vi "Simulation Interface.vi"(8 "error in (no error)":errorcluster, 11 "View Model":T1) -> (0 "error out":errorcluster)   [LabVIEW 2017]
doc: "A program that is run to test Elevator algorithms in a SW-only environment."
uses:
  View Model/Controls/View Model.ctl
  View Model/Controls/Shared Model.ctl
  Error/Controls/Error Model.ctl
  Error/Controls/Error Event.ctl
  Error/Controls/Error Type.ctl
  Configuration/Controls/Config DB Model.ctl
  Configuration/Controls/Config DB Command.ctl
  Configuration/Controls/Config DB Record.ctl
  Controller/Controls/Controller Model.ctl
  Controller/Controls/Elevator Location.ctl
  Controller/Controls/Elevator Direction Event.ctl
  Controller/Controls/Elevator Direction.ctl
  Controller/Controls/Elevator CMD Event.ctl
  Controller/Controls/Elevator Commands.ctl
  Controller/Controls/Elevator Overhead.ctl
  Controller/Controls/Elevator State.ctl
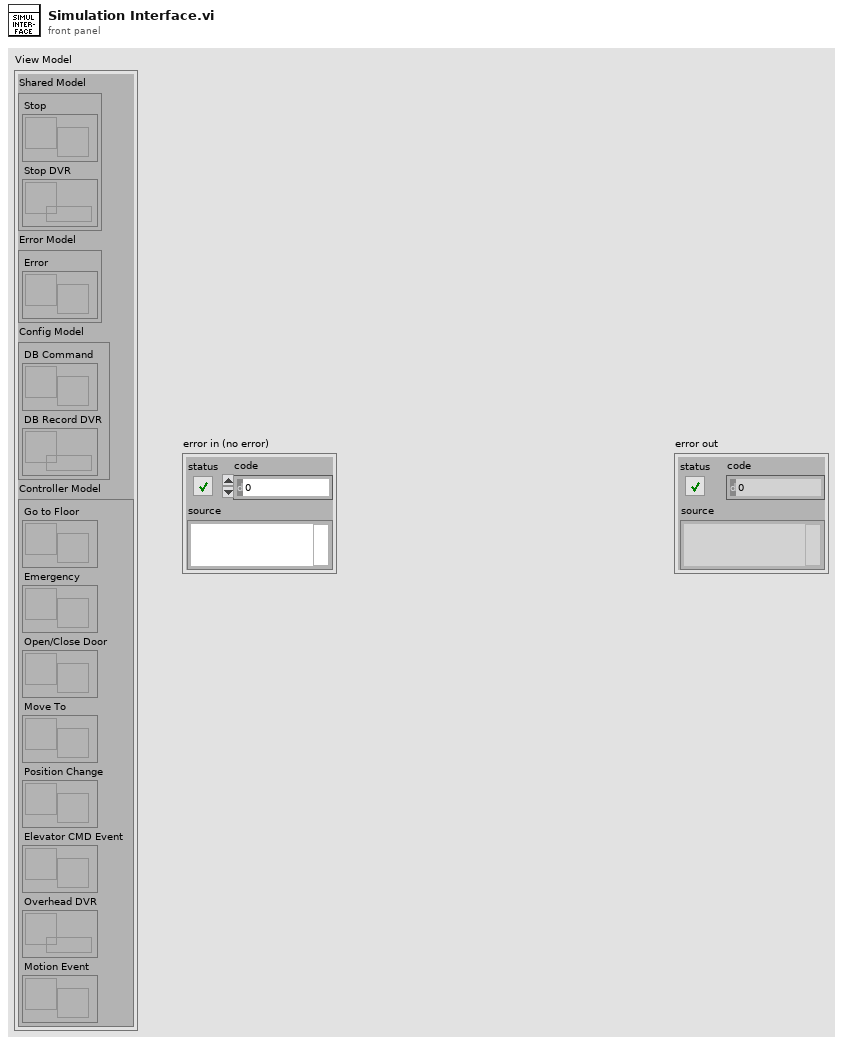
[diagram p1: front panel]
types:
  T1 = typedef "View Model.ctl" = cluster{"Shared Model":T2, "Error Model":T3, "Config Model":T4, "Controller Model":T5}
  T2 = typedef "Shared Model.ctl" = cluster{"Stop":refnum<user-event>, "Stop DVR":refnum<data-value>}
  T3 = typedef "Error Model.ctl" = cluster{"Error":refnum<user-event>}
  T4 = typedef "Config DB Model.ctl" = cluster{"DB Command":refnum<user-event>, "DB Record DVR":refnum<data-value>}
  T5 = typedef "Controller Model.ctl" = cluster{"Go to Floor":refnum<user-event>, "Emergency":refnum<user-event>, "Open/Close Door":refnum<user-event>, "Move To":refnum<user-event>, "Position Change":refnum<user-event>, "Elevator CMD Event":refnum<user-event>, "Overhead DVR":refnum<data-value>, "Motion Event":refnum<user-event>}
  T6 = enum32{"invalid app kind", "Development System", "Run Time System", "Student Edition", "Embedded LabVIEW", "Evaluation", "Custom"}
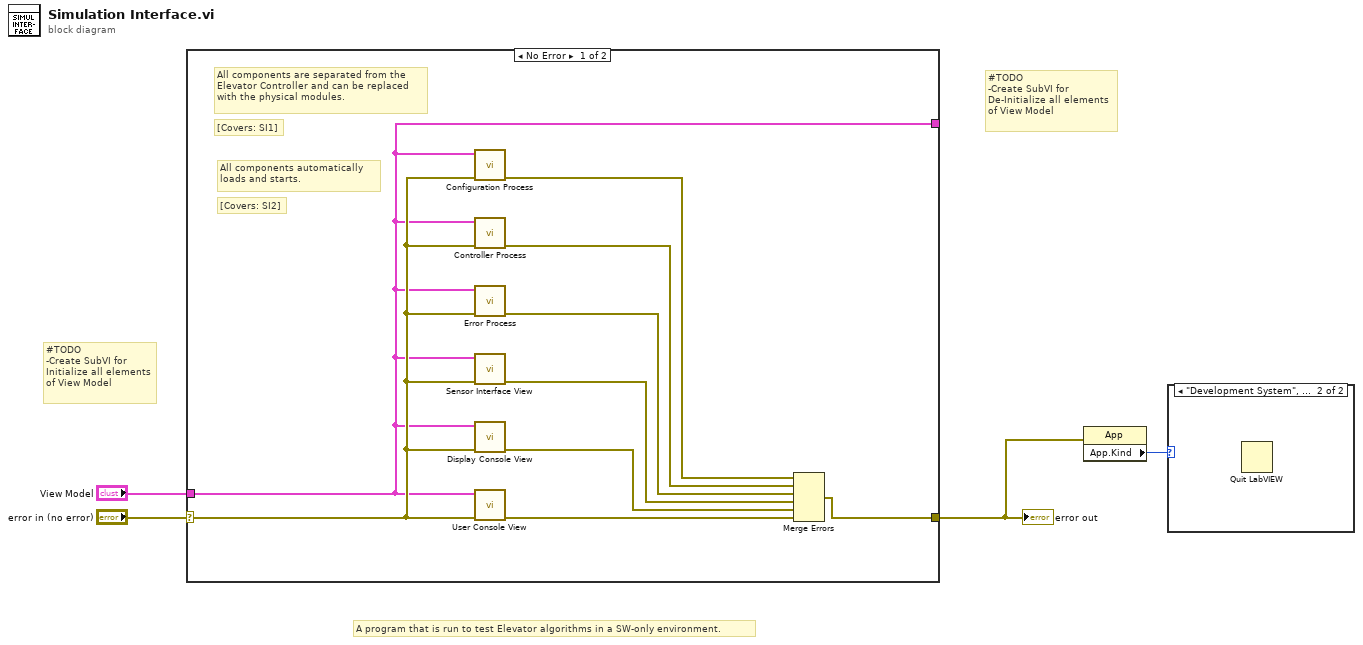
[diagram p0: block diagram]
diagram:
  # "#TODO\n-Create SubVI for\nDe-Initialize all elements\nof View Model"
  # "#TODO\n-Create SubVI for\nInitialize all elements\nof View Model"
  # "A program that is run to test Elevator algorithms in a SW-only environment."
  n1 = case shown="No Error" "error in (no error)" {
    selector: "error in (no error)" -> [w13 w15]
    tunnel: "View Model" -> [w5 w14]
    tunnel: [w6 w15] -> w1
    tunnel: [w5 w14] -> _
    frame No Error {
      # "[Covers: SI2]"
      # "All components automatically\nloads and starts."
      # "[Covers: SI1]"
      # "All components are separated from the \nElevator Controller and can be replaced\nwith the physical modules."
      n2 = call "Configuration Process.vi"("error in (no error)"=w13, "View Model"=w5) -> ("error out"=w7:errorcluster)  [unwired: 9 in]
      n3 = call "Controller Process.vi"("error in (no error)"=w13, "View Model"=w5) -> ("error out"=w8:errorcluster)  [unwired: 9 in]
      n4 = call "Error Process.vi"("error in (no error)"=w13, "View Model"=w5) -> ("error out"=w9:errorcluster)  [unwired: 9 in]
      n5 = call "Sensor Interface View.vi"("error in (no error)"=w13, "View Model"=w5) -> ("error out"=w10:errorcluster)  [unwired: 9 in]
      n6 = call "Display Console View.vi"("error in (no error)"=w13, "View Model"=w5) -> ("error out"=w11:errorcluster)  [unwired: 9 in]
      n7 = call "User Console View.vi"("error in (no error)"=w13, "View Model"=w5) -> ("error out"=w12:errorcluster)  [unwired: 9 in]
      n8 = Merge Errors(w7, w8, w9, w10, w11, w12) -> (w6:errorcluster)
    }
    frame Error {
    }
  }
  "error out" <- w1
  n9 = property class="App"(error in=w1) -> ("App.Kind"=w2:T6)  [unwired: 1 in, 2 out]
  n10 = case shown="\"Development System\", Default" w2 {
    frame "Run Time System" {
    }
    frame "Development System", Default {
      n11 = Quit LabVIEW() -> ()  [unwired: 1 in]
    }
  }
